vi "getData.vi"(8 "error in (no error)":errorcluster, 11 "reference in":refnum<class "checkOUT.lvclass">) -> (0 "error out":errorcluster, 2 "data":string[][](array[string]), 3 "reference out":refnum<class "checkOUT.lvclass">)   [LabVIEW 2016, in "checkOUT.lvclass"]
uses:
  checkOUT.lvclass
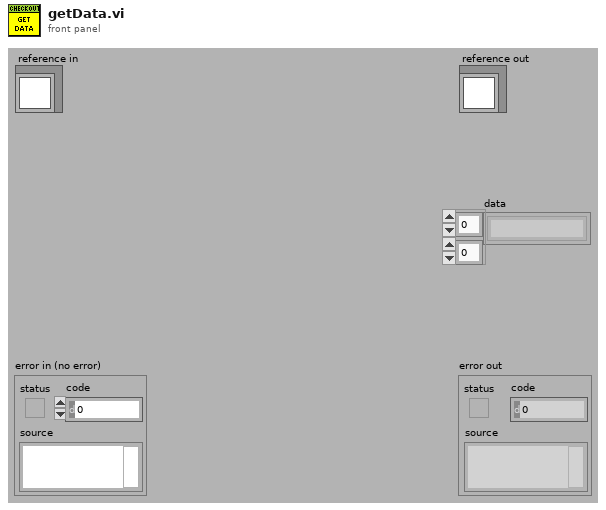
[diagram p1: front panel]
types:
  T1 = typedef "checkOUT.lvclass/ObjectAttributesRef.ctl" = refnum<data-value>
  T2 = typedef "checkOUT.lvclass/ObjectAttributes.ctl" = cluster{"MyAttribute":dbl, "data":string[][]}
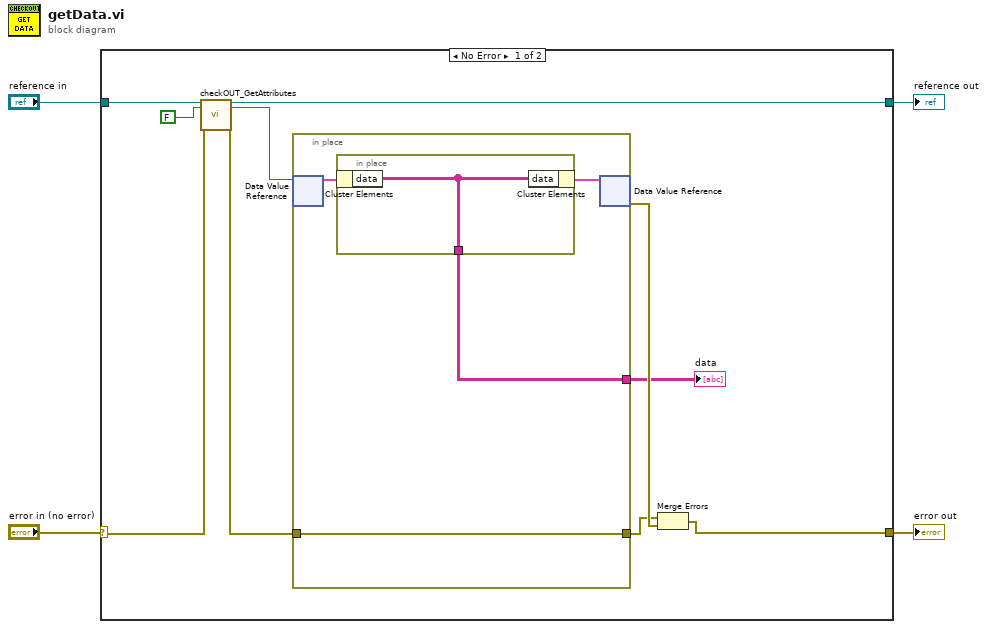
[diagram p0: block diagram]
diagram:
  n1 = case shown="No Error" "error in (no error)" {
    selector: "error in (no error)" -> [w9 w21]
    tunnel: [w14 w21] -> w3
    tunnel: [w7 w20] -> w1
    tunnel: "reference in" -> [w11 w20]
    frame No Error {
      n2 = call "checkOUT_GetAttributes.vi"("reference in"=w11, "return data? (T)"=FALSE, "error in (no error)"=w9) -> ("reference out"=w7:refnum<class "checkOUT.lvclass">, "attributes ref"=w6:T1, "error out"=w8:errorcluster)  [unwired: 13 in, 1 out]
      n3 = in-place {
        in-place-border: w8 -> [w16]
        in-place-border: [w16] -> w12
        in-place-border: [w15] -> w5
        n4 = in-place-dvr #1(w6) -> (w17:T2)  [unwired: 1 out]
        n5 = in-place {
          in-place-border: [w19] -> w15
          n6 = in-place-cluster #2(w17) -> ("data"=w19:string[][])
          n7 = in-place-cluster #2("data"=w19) -> (w18:T2)
        }
        n8 = in-place-dvr #1(w18) -> (w13:errorcluster)  [unwired: 1 out]
      }
      "data" <- w5
      n9 = Merge Errors(w12, w13) -> (w14:errorcluster)
    }
    frame Error {
    }
  }
  "error out" <- w3
  "reference out" <- w1
